vi "OneSensorMagazineLogic.vi"(3 "Outtake Button":bool, 4 "Intake Side Sensor":bool, 5 "Intake Toggle":bool) -> (0 "Magazine Motors":dbl, 1 "Kicker Motors":dbl, 2 "Intake Motors":dbl)   [LabVIEW 2020]
uses:
  MagazineControl.ctl
  TitanLib/Lib/TitanLib.lvlib
panel:
  out "Current State":T1
  in  "Kicker Power":dbl
  in  "Magazine Power":dbl
  in  "Input Power":dbl
  in  "Initial State":T1
  # "Inputs"
  # "Power Levels"
  # "Outputs"
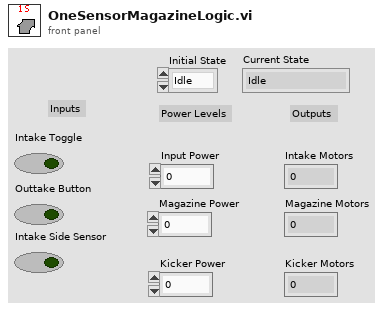
[diagram p1: front panel]
types:
  T1 = typedef "MagazineControl.ctl" = enum16{"Idle", "Intaking", "One Ball", "One Ball Intake", "Two Balls", "Outtake"}
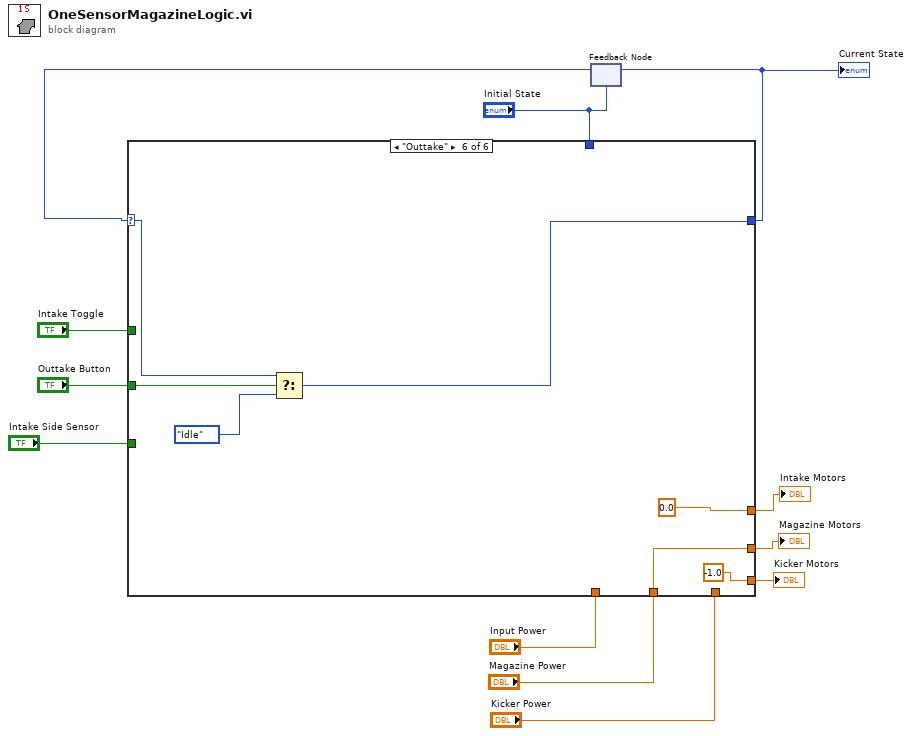
[diagram p0: block diagram]
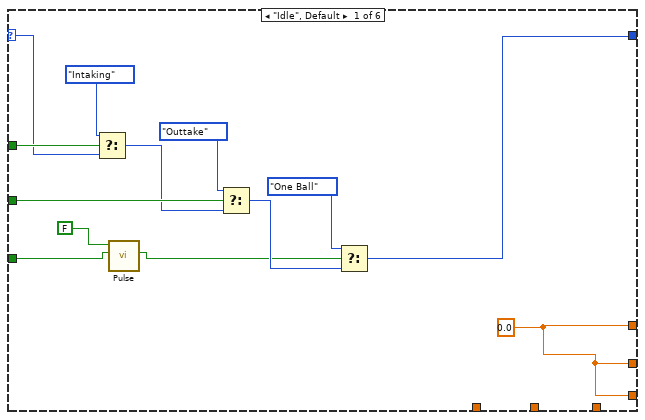
[diagram p2: hidden frame]
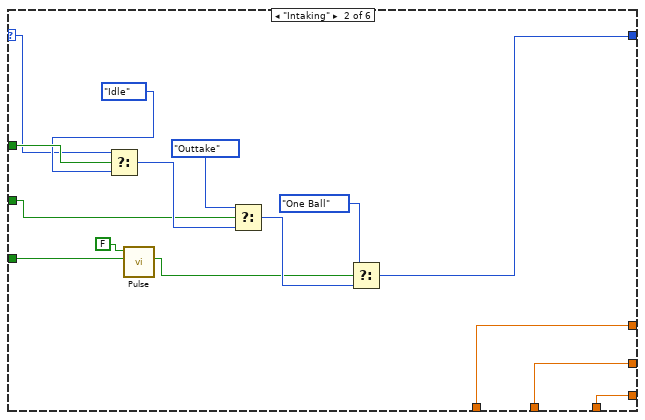
[diagram p3: hidden frame]
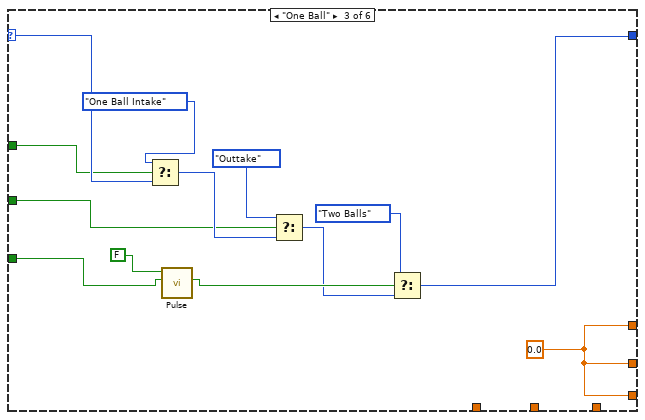
[diagram p4: hidden frame]
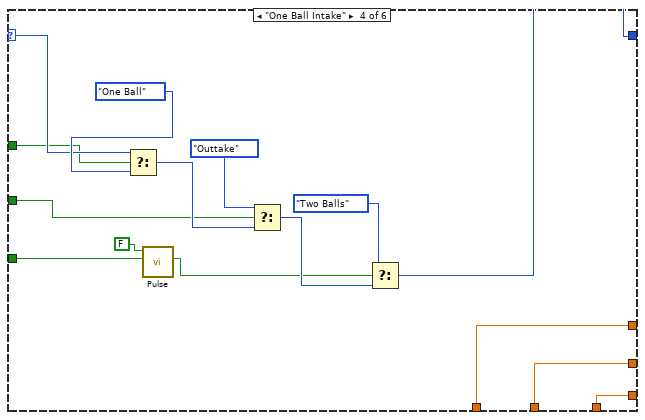
[diagram p5: hidden frame]
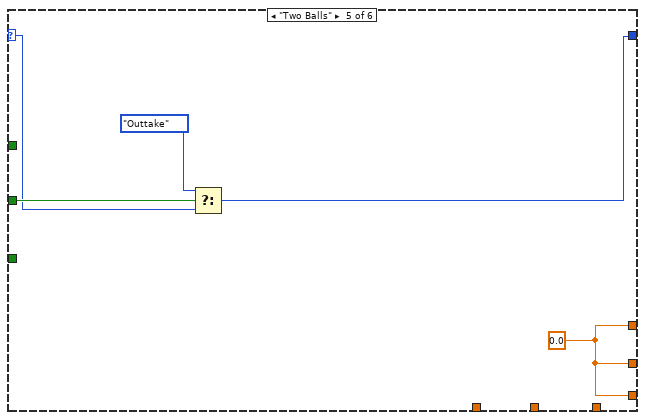
[diagram p6: hidden frame]
diagram:
  n1 = feedback #1("Initial State") -> (w4:T1)
  n2 = case shown="\"Outtake\"" w4 {
    selector: w4 -> [w21 w32 w43 w58 w72 w79]
    tunnel: "Intake Toggle" -> [w25 w35 w42 w57 _ _]
    tunnel: "Outtake Button" -> [w24 w34 w44 w59 w73 w80]
    tunnel: "Intake Side Sensor" -> [w15 w28 w45 w60 _ _]
    tunnel: "Initial State" -> [_ _ _ _ _ _]
    tunnel: [w17 w36 w46 w61 w70 w77] -> w10
    tunnel: [w13 w31 w41 w56 w69 0.0 ("Input Power")] -> w6
    tunnel: "Input Power" -> [_ w31 _ w56 _ _]
    tunnel: [w13 w30 w41 w55 w69 w74] -> w8
    tunnel: "Magazine Power" -> [_ w30 _ w55 _ w74]
    tunnel: [w13 w26 w41 w54 w69 -1.0 ("Kicker Motors")] -> w11
    tunnel: "Kicker Power" -> [_ w26 _ w54 _ _]
    frame "Idle", Default {
      w13 = 0.0 ("Input Power")
      n3 = Select(t=MagazineControl."Intaking", s=w25, f=w21) -> (s? t:f=w23:T1)
      n4 = call "Pulse.vi"("Input"=w15, "Rising Edge?"=FALSE) -> ("Output"=w16:bool)  [unwired: 9 in]
      n5 = Select(t=MagazineControl."Outtake", s=w24, f=w23) -> (s? t:f=w22:T1)
      n6 = Select(t=MagazineControl."One Ball", s=w16, f=w22) -> (s? t:f=w17:T1)
    }
    frame "Intaking" {
      n7 = Select(t=w32, s=w35, f=MagazineControl."Idle" ("t")) -> (s? t:f=w39:T1)
      n8 = call "Pulse.vi"("Input"=w28, "Rising Edge?"=FALSE) -> ("Output"=w29:bool)  [unwired: 9 in]
      n9 = Select(t=MagazineControl."Outtake", s=w34, f=w39) -> (s? t:f=w40:T1)
      n10 = Select(t=MagazineControl."One Ball", s=w29, f=w40) -> (s? t:f=w36:T1)
    }
    frame "One Ball" {
      w41 = 0.0 ("Input Power")
      n11 = Select(t=MagazineControl."One Ball Intake", s=w42, f=w43) -> (s? t:f=w51:T1)
      n12 = call "Pulse.vi"("Input"=w45, "Rising Edge?"=FALSE) -> ("Output"=w53:bool)  [unwired: 9 in]
      n13 = Select(t=MagazineControl."Outtake", s=w44, f=w51) -> (s? t:f=w52:T1)
      n14 = Select(t=MagazineControl."Two Balls", s=w53, f=w52) -> (s? t:f=w46:T1)
    }
    frame "One Ball Intake" {
      n15 = Select(t=w58, s=w57, f=MagazineControl."One Ball" ("t")) -> (s? t:f=w67:T1)
      n16 = call "Pulse.vi"("Input"=w60, "Rising Edge?"=FALSE) -> ("Output"=w63:bool)  [unwired: 9 in]
      n17 = Select(t=MagazineControl."Outtake", s=w59, f=w67) -> (s? t:f=w68:T1)
      n18 = Select(t=MagazineControl."Two Balls", s=w63, f=w68) -> (s? t:f=w61:T1)
    }
    frame "Two Balls" {
      w69 = 0.0 ("Input Power")
      n19 = Select(t=MagazineControl."Outtake", s=w73, f=w72) -> (s? t:f=w70:T1)
    }
    frame "Outtake" {
      n20 = Select(t=w79, s=w80, f=MagazineControl."Idle") -> (s? t:f=w77:T1)
    }
  }
  "Intake Motors" <- w6
  "Magazine Motors" <- w8
  "Kicker Motors" <- w11
  "Current State" <- w10
  n21 = feedback-in #1(w10) -> ()
